vi "Inst_CNT90.vi"(8 "error in":errorcluster, 10 "All Message Queues in":T1, 11 "Prueba31 in":refnum<class "Prueba33.lvclass">) -> (0 "error out":errorcluster)   [LabVIEW 2019, in "Prueba33.lvclass"]
uses:
  Prueba33.lvclass
  QMH/Message Queue/All Message Queues.ctl
  QMH/Message Queue/Message Cluster.ctl
  Prueba33.lvclass/Prueba33.ctl
  <vilib>/Utility/error.llb/Error Cluster From Error Code.vi
  QMH/Message Queue/Enqueue Message (Single).vi
  <vilib>/ErrorRing/Error Ring.xnode
  QMH/Message Queue/Message Queue.lvlib
  Instrumento/CNT90/CNT90.lvclass
panel:
  out "All States":string[](array[string])
  out "Actual State":string
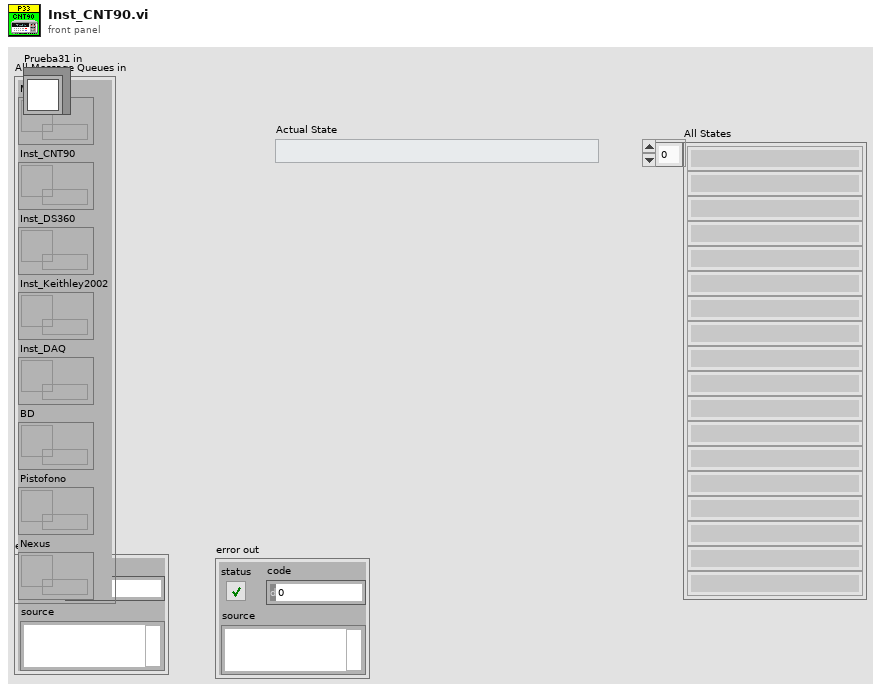
[diagram p1: front panel]
types:
  T1 = typedef "Message Queue.lvlib/All Message Queues.ctl" = cluster{"MHL":refnum<queue>, "Inst_CNT90":refnum<queue>, "Inst_DS360":refnum<queue>, "Inst_Keithley2002":refnum<queue>, "Inst_DAQ":refnum<queue>, "BD":refnum<queue>, "Pistofono":refnum<queue>, "Nexus":refnum<queue>}
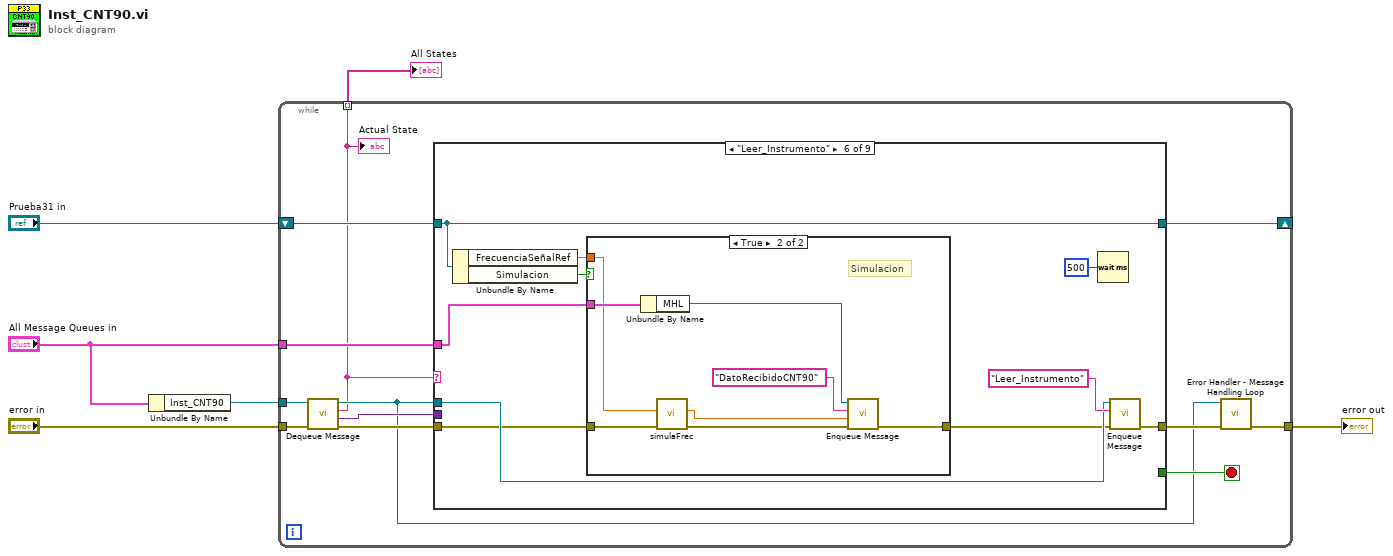
[diagram p0: block diagram]
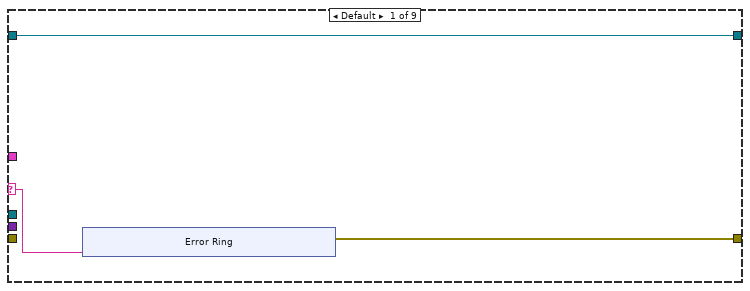
[diagram p2: hidden frame]
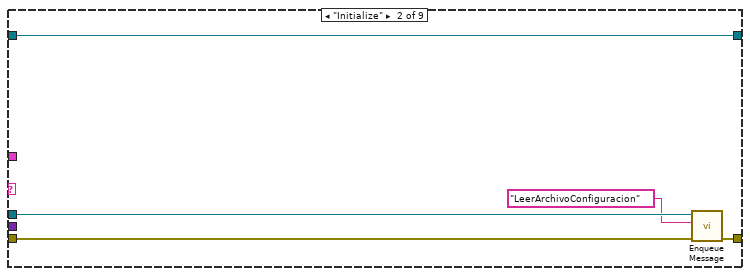
[diagram p3: hidden frame]
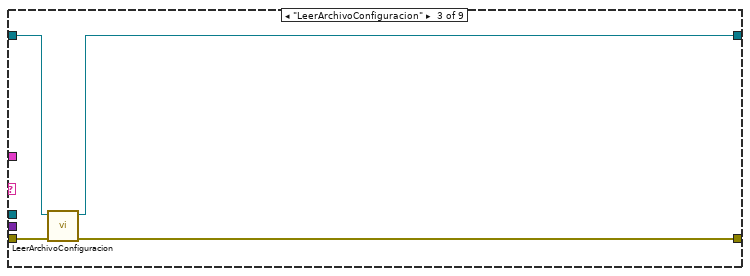
[diagram p4: hidden frame]
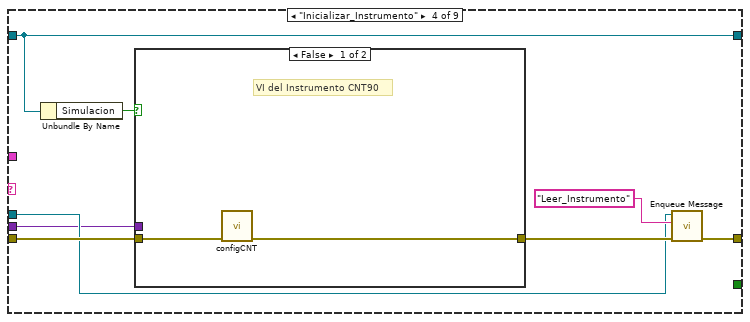
[diagram p5: hidden frame]
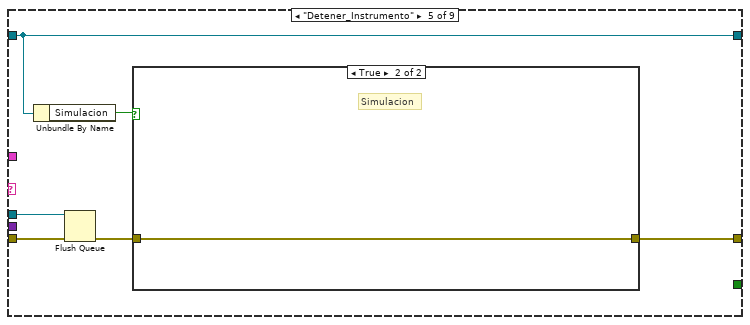
[diagram p7: hidden frame]
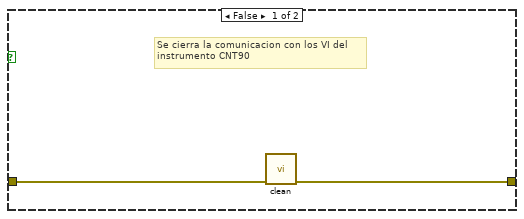
[diagram p8: hidden frame]
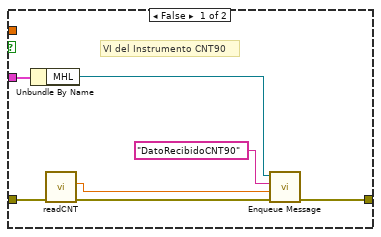
[diagram p9: hidden frame]
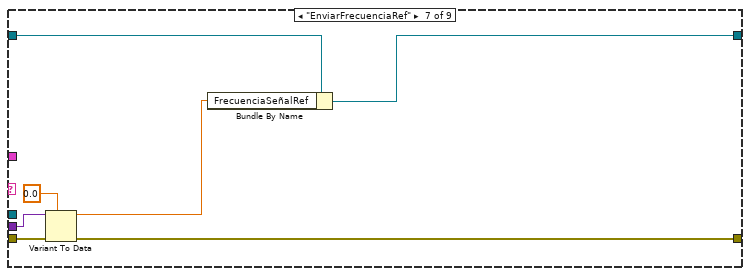
[diagram p10: hidden frame]
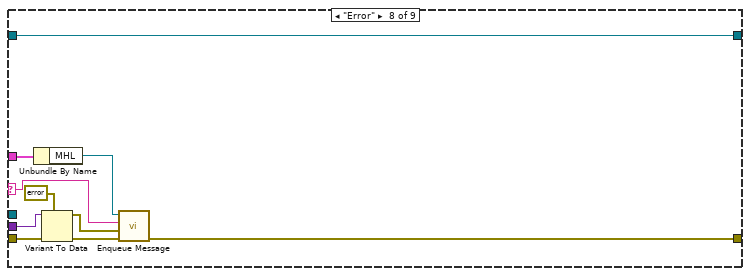
[diagram p11: hidden frame]
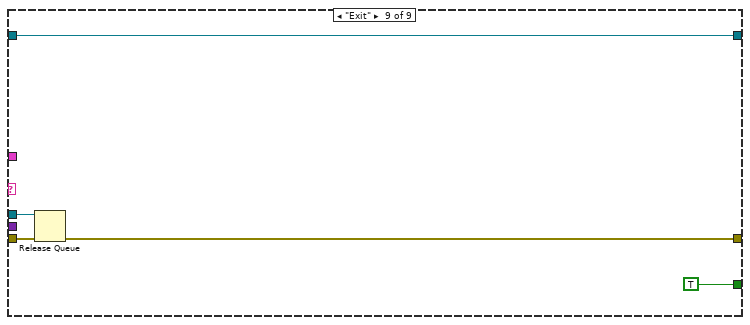
[diagram p12: hidden frame]
diagram:
  n1 = Unbundle By Name("All Message Queues in") -> ("Inst_CNT90"=w4:refnum<queue>)
  n2 = while {
    tunnel: "error in" -> [w18]
    tunnel: w4 -> [w17]
    tunnel: "All Message Queues in" -> [w16]
    tunnel: [w9] -> w2
    shift-right: [w12] -> _
    shift-left: "Prueba31 in" -> [w15]
    tunnel: [w7] -> w1 mode=indexing
    stop <- w11 stop-if-true
    n3 = call "Dequeue Message.vi"("error in (no error)"=w18, "Message Queue"=w17) -> ("error out"=w13:errorcluster, "Message Data"=w14:variant, "Message"=w7:string, "dup Message Queue"=w8:refnum<queue>)  [unwired: 6 in]
    "Actual State" <- w7
    n4 = case shown="\"Leer_Instrumento\"" w7 {
      selector: w7 -> [w21 _ _ _ _ _ _ w94 _]
      tunnel: w16 -> [_ _ _ _ _ w59 _ w93 _]
      tunnel: w15 -> [w19 w33 w35 w45 w53 w61 w84 w91 w101]
      tunnel: w8 -> [_ w30 _ w39 w49 w65 _ _ w103]
      tunnel: w14 -> [_ _ _ w38 _ _ w87 w97 _]
      tunnel: w13 -> [_ w31 w37 w44 w50 w63 w88 w98 w104]
      tunnel: [w20 w32 w34 w41 w54 w66 w89 w90 w100] -> w10
      tunnel: [w19 w33 w36 w45 w53 w61 w85 w91 w101] -> w12
      tunnel: [_ _ _ _ _ _ _ _ TRUE] -> w11
      frame Default {
        n5 = xnode "Error Ring"("parameter 0"=w21) -> ("error out"=w20:errorcluster)
      }
      frame "Initialize" {
        n6 = call-poly "Enqueue Message.vi"("error in (no error)"=w31, "Message"="LeerArchivoConfiguracion", "Message Queue"=w30) -> ("error out"=w32:errorcluster)  [unwired: 7 in, 1 out]
      }
      frame "LeerArchivoConfiguracion" {
        n7 = call "LeerArchivoConfiguracion.vi"("error in"=w37, "Prueba31 in"=w35) -> ("error out"=w34:errorcluster, "Prueba31 out"=w36:refnum<class "Prueba33.lvclass">)  [unwired: 8 in]
      }
      frame "Inicializar_Instrumento" {
        n8 = Unbundle By Name(w45) -> ("Simulacion"=w43:bool)
        n9 = case shown="False" w43 {
          tunnel: [w47 w48] -> w40
          tunnel: w44 -> [w46 w48]
          tunnel: w38 -> [_ _]
          frame False {
            # "VI del Instrumento CNT90"
            n10 = call "configCNT.vi"("error in (no error)"=w46) -> ("error out"=w47:errorcluster)  [unwired: 9 in, 1 out]
          }
          frame True {
            # "Simulacion"
          }
        }
        n11 = call-poly "Enqueue Message.vi"("error in (no error)"=w40, "Message"="Leer_Instrumento", "Message Queue"=w39) -> ("error out"=w41:errorcluster)  [unwired: 7 in, 1 out]
      }
      frame "Detener_Instrumento" {
        n12 = Unbundle By Name(w53) -> ("Simulacion"=w52:bool)
        n13 = Flush Queue(queue=w49, error in (no error)=w50) -> (error out=w51:errorcluster)  [unwired: 2 out]
        n14 = case shown="True" w52 {
          tunnel: [w56 w57] -> w54
          tunnel: w51 -> [w55 w57]
          frame False {
            # "Se cierra la comunicacion con los VI del\ninstrumento CNT90"
            n15 = call "clean.vi"("error in (no error)"=w55) -> ("error out"=w56:errorcluster)  [unwired: 9 in, 1 out]
          }
          frame True {
            # "Simulacion"
          }
        }
      }
      frame "Leer_Instrumento" {
        n16 = Unbundle By Name(w61) -> ("FrecuenciaSeñalRef"=w58:dbl, "Simulacion"=w60:bool)
        n17 = case shown="True" w60 {
          tunnel: [w71 w81] -> w62
          tunnel: w63 -> [w74 w78]
          tunnel: w59 -> [w70 w80]
          tunnel: w58 -> [_ w75]
          frame False {
            # "VI del Instrumento CNT90"
            n18 = Unbundle By Name(w70) -> ("MHL"=w69:refnum<queue>)
            n19 = call "readCNT.vi"("error in (no error)"=w74) -> ("error out"=w72:errorcluster, "medicion"=w68:dbl)  [unwired: 8 in, 1 out]
            n20 = call-poly "Enqueue Message.vi"("error in (no error)"=w72, "Message Data"=w68, "Message"="DatoRecibidoCNT90", "Message Queue"=w69) -> ("error out"=w71:errorcluster)  [unwired: 6 in, 1 out]
          }
          frame True {
            # "Simulacion"
            n21 = Unbundle By Name(w80) -> ("MHL"=w79:refnum<queue>)
            n22 = call "simulaFrec.vi"("error in (no error)"=w78, "frec in"=w75) -> ("error out"=w77:errorcluster, "frec out"=w76:dbl)  [unwired: 7 in, 1 out]
            n23 = call-poly "Enqueue Message.vi"("error in (no error)"=w77, "Message Data"=w76, "Message"="DatoRecibidoCNT90", "Message Queue"=w79) -> ("error out"=w81:errorcluster)  [unwired: 6 in, 1 out]
          }
        }
        n24 = Wait (ms)(milliseconds to wait=u32 500) -> ()  [unwired: 1 out]
        n25 = call-poly "Enqueue Message.vi"("error in (no error)"=w62, "Message"="Leer_Instrumento", "Message Queue"=w65) -> ("error out"=w66:errorcluster)  [unwired: 7 in, 1 out]
      }
      frame "EnviarFrecuenciaRef" {
        n26 = Variant To Data(error in=w88, type=0.0, Variant=w87) -> (data=w83:dbl, error out=w89:errorcluster)
        n27 = Bundle By Name(cluster=w84, "FrecuenciaSeñalRef"=w83) -> (w85:refnum<class "Prueba33.lvclass">)
      }
      frame "Error" {
        n28 = Unbundle By Name(w93) -> ("MHL"=w92:refnum<queue>)
        n29 = Variant To Data(error in=w98, type=errorcluster {"status"=FALSE, "code"=0, "source"=""} ("error constant"), Variant=w97) -> (data=w95:errorcluster, error out=w96:errorcluster)
        n30 = call-poly "Enqueue Message.vi"("error in (no error)"=w96, "Message Data"=w95, "Message"=w94, "Message Queue"=w92) -> ("error out"=w90:errorcluster)  [unwired: 6 in, 1 out]
      }
      frame "Exit" {
        n31 = Release Queue(queue=w103, error in (no error)=w104) -> (error out=w100:errorcluster)  [unwired: 1 in, 2 out]
      }
    }
    n32 = call "Error Handler - Message Handling Loop.vi"("error in (no error)"=w10, "Message Queue"=w8) -> ("dup error in"=w9:errorcluster)  [unwired: 8 in, 1 out]
  }
  "error out" <- w2
  "All States" <- w1
